vi "Actor Core.vi"(8 "error in":errorcluster, 11 "Iterator Actor in":refnum<class "Iterator Actor.lvclass">) -> (0 "error out":errorcluster, 3 "Actor out":refnum<class "Actor.lvclass">)   [LabVIEW 2017, in "Iterator Actor.lvlib" / "Iterator Actor.lvclass"]
doc: "(<B>Filename</B>: Actor Framework.lvlib:Actor.lvclass:Actor Core.vi)\n\nReceives messages to the actor, reacts to them, and initiates any error handling that may shut the actor down.\n\nDescendant classes may override this VI to append parallel tasks for the actor to complete while it handles messages. Overrides use the Call Parent Method node."
uses:
  Iterator Actor.lvclass
  C:/Program Files (x86)/National Instruments/LabVIEW 2017/vi.lib/ActorFramework/Actor/Actor.lvclass
  <vilib>/ActorFramework/Actor/Actor.lvclass
  <vilib>/ActorFramework/Actor/Actor.lvclass/Actor.ctl
  <vilib>/ActorFramework/Message Enqueuer/Message Enqueuer.lvclass/Message Enqueuer.ctl
  Iterator Actor.lvclass/Iterator Actor.ctl
  Iterator Settings.ctl
  Stop Condition.ctl
  Iterator Actor Abstract Messages/Iterator Reply Msg/Iterator Reply Msg.lvclass
  Iterator Actor Abstract Messages/Iterator Report Error Msg/Iterator Report Error Msg.lvclass
  <vilib>/ActorFramework/Message Enqueuer/Init from Existing Queue.vi
  <vilib>/ActorFramework/Message Enqueuer/Message Enqueuer.lvclass
  Iterator Actor Messages/Report Errors Msg/Report Errors Msg.lvclass
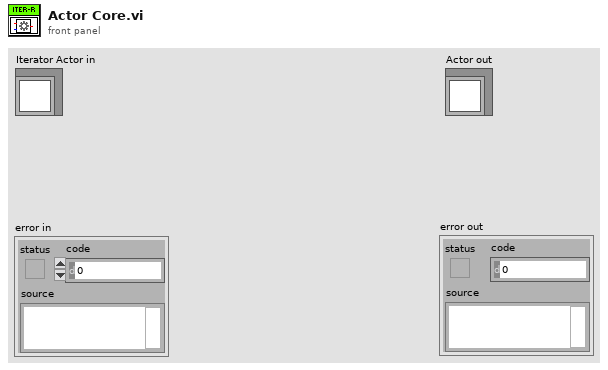
[diagram p1: front panel]
types:
  T1 = typedef "Iterator Actor.lvlib/Iterator Actor.lvclass/Iterator Settings.ctl" = cluster{"Prepare timeout (ms)":i32, "Iterate timeout (ms)":i32, "Conclude timeout (ms)":i32, "Iterate period (ms)":i32, "Number of iterations":i32, "Stop Condition":T2, "Time before stop (ms)":i32, "Prepare Msg":refnum<class "Iterator Reply Msg.lvclass">, "Iterate Msg":refnum<class "Iterator Reply Msg.lvclass">, "Conclude Msg":refnum<class "Iterator Reply Msg.lvclass">, "Error Handler":refnum<class "Iterator Report Error Msg.lvclass">}
  T2 = typedef "Iterator Actor.lvlib/Iterator Actor.lvclass/Stop Condition.ctl" = enum16{"None", "Number of Iterations", "Time Elapsed", "Iteration Result"}
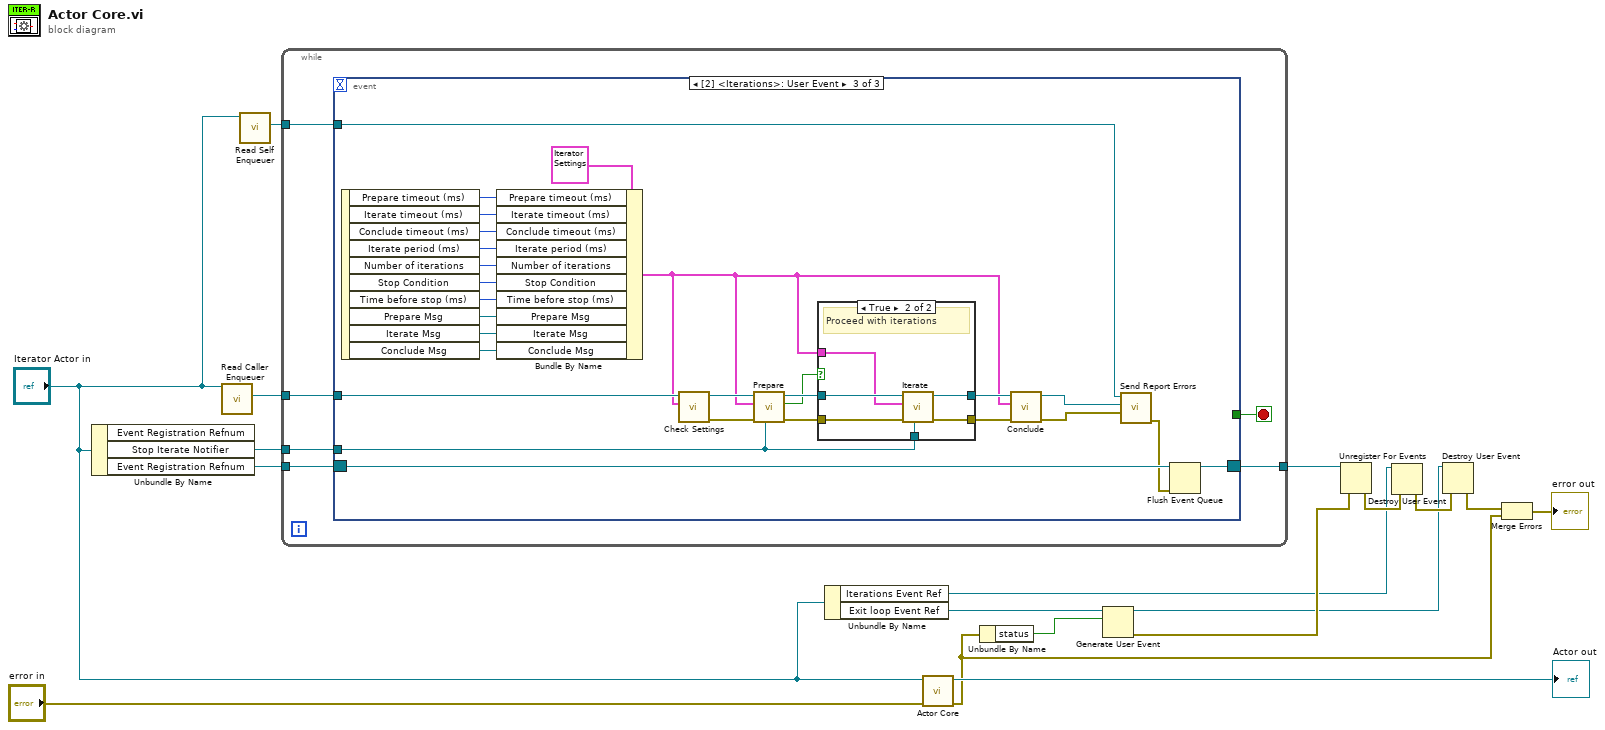
[diagram p0: block diagram]
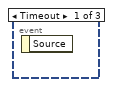
[diagram p2: hidden frame]
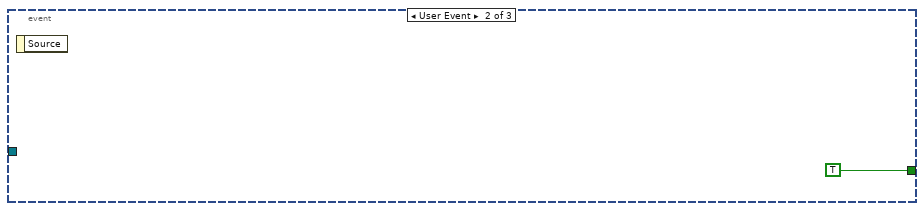
[diagram p3: hidden frame]
diagram:
  n1 = Unbundle By Name("Iterator Actor in") -> ("Stop Iterate Notifier"=w16:refnum<notifier>, "Event Registration Refnum"=w3:refnum<event-registration>)  [unwired: 1 out]
  n2 = call <vilib>:"Read Caller Enqueuer.vi"("Actor"="Iterator Actor in") -> ("Caller Enqueuer"=w17:refnum<class "Message Enqueuer.lvclass">)  [unwired: 10 in]
  n3 = call <vilib>:"Read Self Enqueuer.vi"("Actor"="Iterator Actor in") -> ("Self Enqueuer"=w1:refnum<class "Message Enqueuer.lvclass">)  [unwired: 10 in]
  n4 = while {
    tunnel: w3 -> [w24]
    tunnel: w17 -> [w23]
    tunnel: w16 -> [w21]
    tunnel: [w20] -> w13
    tunnel: w1 -> [w19]
    stop <- w22 stop-if-true
    n5 = event shown="[2] <Iterations>: User Event" {
      selector: w24 -> [_ _ w31]
      dyn-events: [_ _ w32] -> w20
      timeout: _ -> [_ _ _]
      tunnel: w23 -> [_ _ w36]
      tunnel: [_ TRUE _] -> w22
      tunnel: w21 -> [_ _ w30]
      tunnel: w19 -> [_ _ w28]
      event Timeout {
        n6 = event-data() -> ()  [unwired: 1 in, 1 out]
      }
      event User Event {
        n7 = event-data() -> ()  [unwired: 1 in, 1 out]
      }
      event User Event {
        n8 = event-data() -> ("Prepare timeout (ms)"=w50:i32, "Iterate timeout (ms)"=w49:i32, "Conclude timeout (ms)"=w48:i32, "Iterate period (ms)"=w47:i32, "Number of iterations"=w46:i32, "Stop Condition"=w45:T2, "Time before stop (ms)"=w44:i32, "Prepare Msg"=w43:refnum<class "Iterator Reply Msg.lvclass">, "Iterate Msg"=w42:refnum<class "Iterator Reply Msg.lvclass">, "Conclude Msg"=w41:refnum<class "Iterator Reply Msg.lvclass">)  [unwired: 1 in]
        n9 = Bundle By Name(cluster=T1 {"Prepare timeout (ms)"=0, "Iterate timeout (ms)"=0, "Conclude timeout (ms)"=0, "Iterate period (ms)"=0, "Number of iterations"=0, "Stop Condition"=enum."None", "Time before stop (ms)"=0, "Prepare Msg"=refnum, "Iterate Msg"=refnum, "Conclude Msg"=refnum, "Error Handler"=refnum} ("Iterator Settings"), "Prepare timeout (ms)"=w50, "Iterate timeout (ms)"=w49, "Conclude timeout (ms)"=w48, "Iterate period (ms)"=w47, "Number of iterations"=w46, "Stop Condition"=w45, "Time before stop (ms)"=w44, "Prepare Msg"=w43, "Iterate Msg"=w42, "Conclude Msg"=w41) -> (w33:T1)
        n10 = call "Check Settings.vi"("Iterator Settings"=w33, "Caller Enqueuer in"=w36) -> ("error out"=w34:errorcluster, "Caller Enqueuer out"=w35:refnum<class "Message Enqueuer.lvclass">)  [unwired: 8 in]
        n11 = call "Prepare.vi"("notifier in"=w30, "error in"=w34, "Iterator Settings"=w33, "Caller Enqueuer in"=w35) -> ("error out"=w37:errorcluster, "Reply"=w38:bool, "Caller Enqueuer out"=w40:refnum<class "Message Enqueuer.lvclass">)  [unwired: 5 in]
        n12 = case shown="True" w38 {
          tunnel: w30 -> [_ w57]
          tunnel: [w53 w60] -> w52
          tunnel: w33 -> [_ w55]
          tunnel: w40 -> [w54 w59]
          tunnel: [w54 w58] -> w39
          tunnel: w37 -> [w53 w56]
          frame False {
            # "Do not proceed \nwith iterations"
          }
          frame True {
            # "Proceed with iterations"
            n13 = call "Iterate.vi"("notifier in"=w57, "error in (no error)"=w56, "Iterator Settings"=w55, "Caller Enqueuer in"=w59) -> ("error out"=w60:errorcluster, "Caller Enqueuer out"=w58:refnum<class "Message Enqueuer.lvclass">)  [unwired: 6 in]
          }
        }
        n14 = call "Conclude.vi"("error in (no error)"=w52, "Iterator Settings"=w33, "Caller Enqueuer in"=w39) -> ("error out"=w26:errorcluster, "Caller Enqueuer out"=w29:refnum<class "Message Enqueuer.lvclass">)  [unwired: 7 in]
        n15 = call "Send Report Errors.vi"("Iterator Error"=w26, "Caller Enqueuer in"=w29, "Message Enqueuer in"=w28) -> ("error out"=w27:errorcluster)  [unwired: 7 in, 1 out]
        n16 = Flush Event Queue(0:w31, 3:w27) -> (8:w32:refnum<event-registration>)  [unwired: 4 in, 2 out]
      }
    }
  }
  n17 = Unbundle By Name("Iterator Actor in") -> ("Iterations Event Ref"=w7:refnum<user-event>, "Exit loop Event Ref"=w15:refnum<user-event>)
  n18 = call-parent "Actor Core.vi"("error in"="error in", "Actor in"="Iterator Actor in") -> ("error out"=w5:errorcluster, "Actor out"=→"Actor out":refnum<class "Actor.lvclass">)  [unwired: 8 in]
  n19 = Unbundle By Name(w5) -> ("status"=w4:bool)
  n20 = Generate User Event(user event=w15, event data cluster=w4) -> (user event out=w8:refnum<user-event>, error out=w11:errorcluster)  [unwired: 2 in]
  n21 = Unregister For Events(event registration refnum=w13, error in=w11) -> (error out=w12:errorcluster)
  n22 = Destroy User Event(user event=w7, error in=w12) -> (error out=w10:errorcluster)
  n23 = Destroy User Event(user event=w8, error in=w10) -> (error out=w9:errorcluster)
  n24 = Merge Errors(w9, w5) -> (→"error out":errorcluster)
